vi "prod_year_amee.vi"(8 "Selected Year":string="ST1_PRODUCTION_COUNT", 9 "Station":string(combo), 10 "Shift":string="1", 11 "connection reference":T1) -> (0 "transposed array":string[][](array[string]), 1 "Array":i32[](array[numeric]), 2 "All 2":string[](array[string]), 3 "Array 3":i32[][](array[numeric]))   [LabVIEW 2017]
uses:
  <vilib>/addons/database/Connection.llb/Conn ObjectReference.ctl
  <vilib>/addons/database/Connection.llb/Conn Execute.vi
  <vilib>/addons/database/Recordset.llb/Rec Fetch Recordset Data (R).vi
  <vilib>/addons/database/NI_Database_API.lvlib
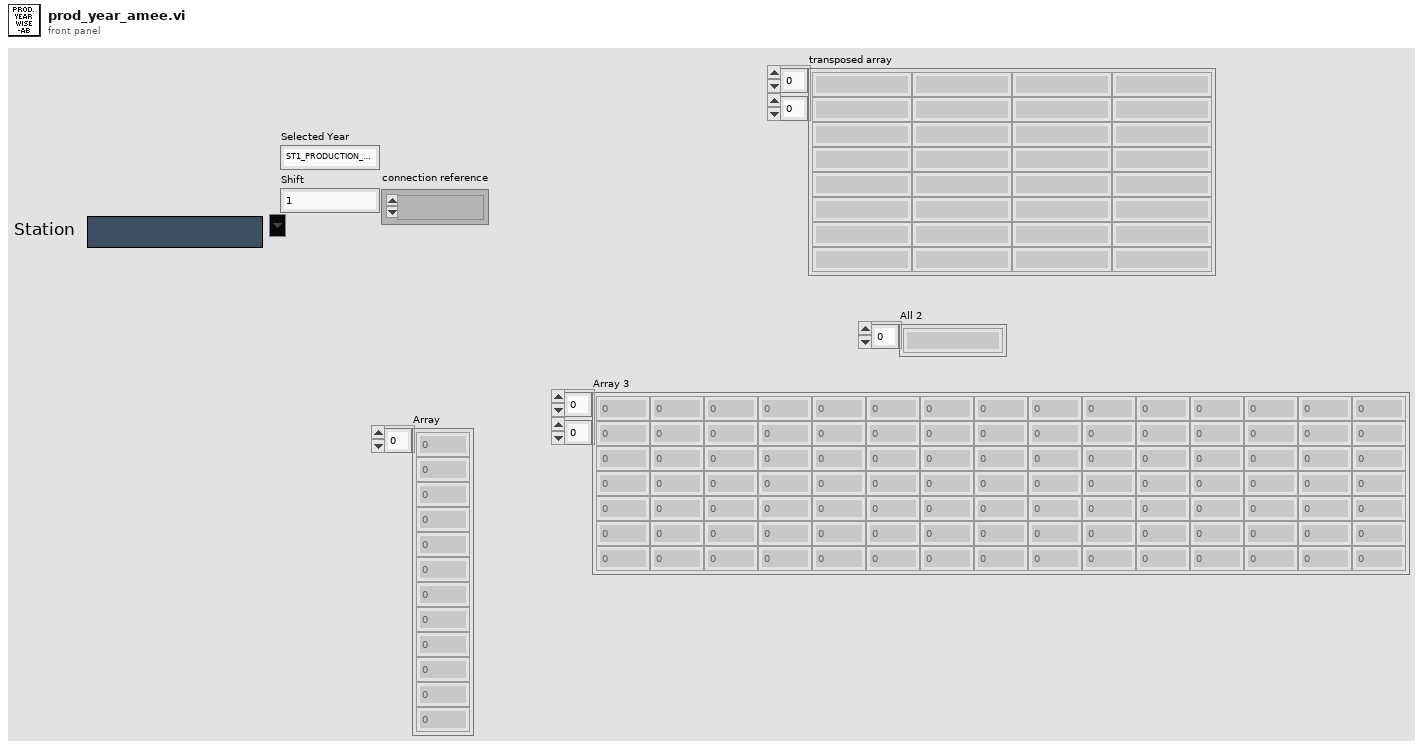
[diagram p1: front panel]
types:
  T1 = typedef "NI_Database_API.lvlib/Conn ObjectReference.ctl" = refnum<k1>
  T2 = typedef "NI_Database_API.lvlib/Rec ObjectReference.ctl" = refnum<k1>
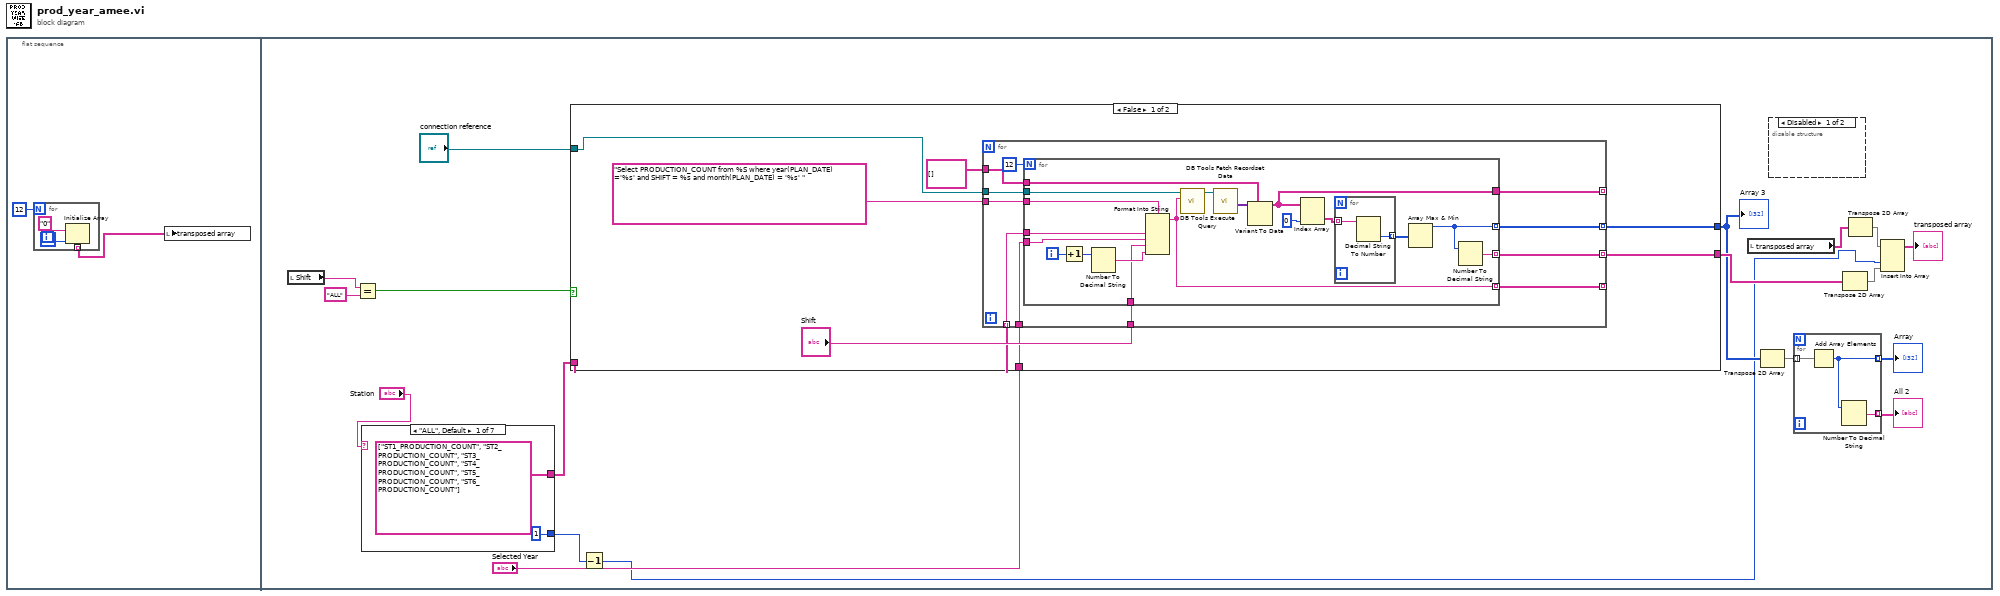
[diagram p0: block diagram]
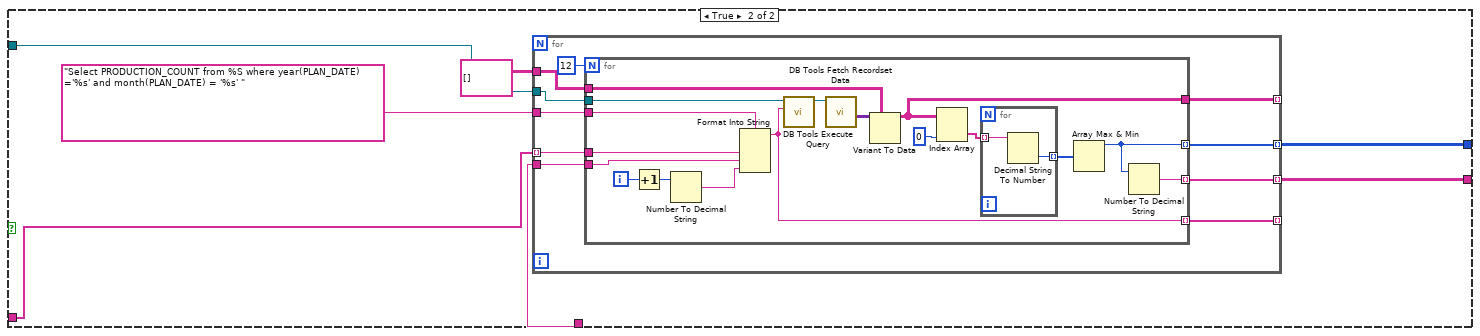
[diagram p3: hidden frame]
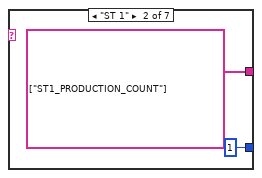
[diagram p4: hidden frame]
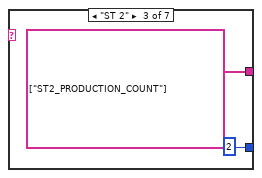
[diagram p5: hidden frame]
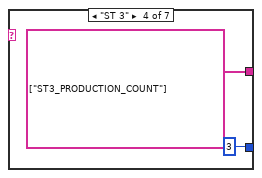
[diagram p6: hidden frame]
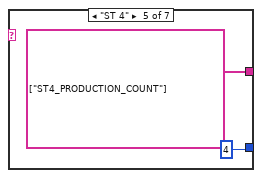
[diagram p7: hidden frame]
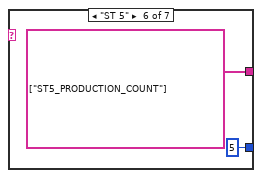
[diagram p8: hidden frame]
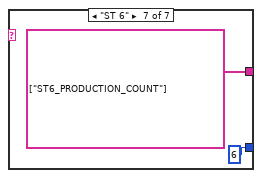
[diagram p9: hidden frame]
diagram:
  n1 = flat-sequence {
    frame #0 {
      n2 = for {
        N: 12 -> [_]
        tunnel: [w3] -> w2 mode=indexing
        n3 = Initialize Array("0" ("String"), 12 ("dimension size")) -> (w3:string[])
      }
      n4 = local write "transposed array"(w2) -> ()
    }
    frame #1 {
      n5 = local read "Shift"() -> (w23:string)
      n6 = Equal?(x=w23, y="ALL") -> (x = y?=w21:bool)
      n7 = case shown="\"ALL\", Default" "Station" {
        tunnel: [string[] ["ST1_PRODUCTION_COUNT", "ST2_PRODUCTION_COUNT", "ST3_PRODUCTION_COUNT", "ST4_PRODUCTION_COUNT", "ST5_PRODUCTION_COUNT", "ST6_PRODUCTION_COUNT"] string[] ["ST1_PRODUCTION_COUNT"] string[] ["ST2_PRODUCTION_COUNT"] string[] ["ST3_PRODUCTION_COUNT"] string[] ["ST4_PRODUCTION_COUNT"] string[] ["ST5_PRODUCTION_COUNT"] string[] ["ST6_PRODUCTION_COUNT"]] -> w12
        tunnel: [1 1 2 3 4 5 6] -> w7
        frame "ALL", Default {
        }
        frame "ST 1" {
        }
        frame "ST 2" {
        }
        frame "ST 3" {
        }
        frame "ST 4" {
        }
        frame "ST 5" {
        }
        frame "ST 6" {
        }
      }
      n8 = case shown="False" w21 {
        tunnel: "Selected Year" -> [w31 w70]
        tunnel: [w30 w69] -> w17
        tunnel: [w29 w68] -> w19
        tunnel: "connection reference" -> [w28 w67]
        tunnel: w12 -> [w27 w66]
        frame False {
          n9 = for {
            tunnel: "Select PRODUCTION_COUNT from %S where year(PLAN_DATE) ='%s' and SHIFT = %s and month(PLAN_DATE) = '%s' " ("format string") -> [w45]
            tunnel: [w44] -> _ mode=indexing
            tunnel: w28 -> [w43]
            tunnel: string[][] [] -> [w42]
            tunnel: [w41] -> _ mode=indexing
            tunnel: [w36] -> w30 mode=indexing
            tunnel: "Shift" -> [w39]
            tunnel: w31 -> [w38]
            tunnel: [w37] -> w29 mode=indexing
            tunnel: w27 -> [w35] mode=indexing
            n10 = for {
              N: 12 -> [_]
              tunnel: w45 -> [w63]
              tunnel: w35 -> [w62]
              tunnel: w38 -> [w61]
              tunnel: [w57] -> w44 mode=indexing
              tunnel: w43 -> [w56]
              tunnel: w42 -> [w54]
              tunnel: [w52] -> w41
              tunnel: [w47] -> w36 mode=indexing
              tunnel: w39 -> [w48]
              tunnel: [w46] -> w37 mode=indexing
              i -> [w60]
              n11 = Increment(x=w60) -> (x+1=w59:i32)
              n12 = Number To Decimal String(number=w59) -> (decimal integer string=w58:string)  [unwired: 1 in]
              n13 = Format Into String(format string=w63, w62, w61, w48, w58) -> (resulting string=w57:string)  [unwired: 2 in, 1 out]
              n14 = call-poly <vilib>:"DB Tools Execute Query.vi"("SQL query"=w57, "connection reference"=w56) -> ("recordset reference"=w55:T2)  [unwired: 6 in, 1 out]
              n15 = call-poly <vilib>:"DB Tools Fetch Recordset Data.vi"("recordset reference"=w55) -> ("recordset data"=w53:variant[][])  [unwired: 4 in, 2 out]
              n16 = Variant To Data(type=w54, Variant=w53) -> (data=w52:string[][])  [unwired: 1 in, 1 out]
              n17 = Index Array(array=w52, index (col)=0 ("disabled index (col)")) -> (element=w50:string[])  [unwired: 1 in]
              n18 = for {
                tunnel: w50 -> [w65] mode=indexing
                tunnel: [w64] -> w49 mode=indexing
                n19 = Decimal String To Number(string=w65) -> (number=w64:i32)  [unwired: 2 in, 1 out]
              }
              n20 = Array Max & Min(array=w49) -> (max value=w47:i32)  [unwired: 3 out]
              n21 = Number To Decimal String(number=w47) -> (decimal integer string=w46:string)  [unwired: 1 in]
            }
          }
        }
        frame True {
          n22 = for {
            tunnel: "Select PRODUCTION_COUNT from %S where year(PLAN_DATE) ='%s' and month(PLAN_DATE) = '%s' " ("format string") -> [w82]
            tunnel: w66 -> [w81] mode=indexing
            tunnel: w70 -> [w80]
            tunnel: [w79] -> _ mode=indexing
            tunnel: string[][] [] -> [w78]
            tunnel: [w77] -> _ mode=indexing
            tunnel: [w74] -> w69 mode=indexing
            tunnel: [w75] -> w68 mode=indexing
            tunnel: w67 -> [w73]
            n23 = for {
              N: 12 -> [_]
              tunnel: w82 -> [w99]
              tunnel: w81 -> [w98]
              tunnel: w80 -> [w97]
              tunnel: [w93] -> w79 mode=indexing
              tunnel: w78 -> [w91]
              tunnel: [w89] -> w77
              tunnel: [w84] -> w74 mode=indexing
              tunnel: w73 -> [w85]
              tunnel: [w83] -> w75 mode=indexing
              i -> [w96]
              n24 = Increment(x=w96) -> (x+1=w95:i32)
              n25 = Number To Decimal String(number=w95) -> (decimal integer string=w94:string)  [unwired: 1 in]
              n26 = Format Into String(format string=w99, w98, w97, w94) -> (resulting string=w93:string)  [unwired: 2 in, 1 out]
              n27 = call-poly <vilib>:"DB Tools Execute Query.vi"("SQL query"=w93, "connection reference"=w85) -> ("recordset reference"=w92:T2)  [unwired: 6 in, 1 out]
              n28 = call-poly <vilib>:"DB Tools Fetch Recordset Data.vi"("recordset reference"=w92) -> ("recordset data"=w90:variant[][])  [unwired: 4 in, 2 out]
              n29 = Variant To Data(type=w91, Variant=w90) -> (data=w89:string[][])  [unwired: 1 in, 1 out]
              n30 = Index Array(array=w89, index (col)=0 ("disabled index (col)")) -> (element=w87:string[])  [unwired: 1 in]
              n31 = for {
                tunnel: w87 -> [w101] mode=indexing
                tunnel: [w100] -> w86 mode=indexing
                n32 = Decimal String To Number(string=w101) -> (number=w100:i32)  [unwired: 2 in, 1 out]
              }
              n33 = Array Max & Min(array=w86) -> (max value=w84:i32)  [unwired: 3 out]
              n34 = Number To Decimal String(number=w84) -> (decimal integer string=w83:string)  [unwired: 1 in]
            }
          }
        }
      }
      "Array 3" <- w17
      n35 = Decrement(x=w7) -> (x-1=w6:i32)
      n36 = local read "transposed array"() -> (w9:string[][])
      n37 = Transpose 2D Array(2D array=w17) -> (transposed array=w16:i32[][])
      n38 = disable-structure shown="Disabled" {
        frame Disabled {
        }
        frame Enabled {
        }
      }
      n39 = for {
        tunnel: w16 -> [w26] mode=indexing
        tunnel: [w24] -> w18 mode=indexing
        tunnel: [w25] -> w15 mode=indexing
        n40 = Add Array Elements(numeric array=w26) -> (sum=w24:i32)
        n41 = Number To Decimal String(number=w24) -> (decimal integer string=w25:string)  [unwired: 1 in]
      }
      "Array" <- w18
      "All 2" <- w15
      n42 = Transpose 2D Array(2D array=w19) -> (transposed array=w10:string[][])
      n43 = Transpose 2D Array(2D array=w9) -> (transposed array=w8:string[][])
      n44 = Insert Into Array(array=w8, index (col)=w6, new element=w10) -> (→"transposed array":string[][])  [unwired: 1 in]
    }
  }
